vi "XY Graph Check-Uncheck Menu Items.vi"(8 "Error In":errorcluster, 10 "Menu in":refnum<k9>, 11 "XY Graph Refnum":T1) -> (0 "Error Out (dup)":errorcluster, 1 "Click Location":T2, 2 "Menu out":refnum<k9>, 3 "XY Graph Refnum dup":T1)   [LabVIEW 2021, in "XY Graph Add-Ons.lvlib"]
doc: "Check whether the Tools Panels and Grida are visible or not, and add/remove checkmarks accordingly."
uses:
  XY Graph Add-Ons.lvlib
  XY Graph Refnum.ctl
  XY Graph Click Location.ctl
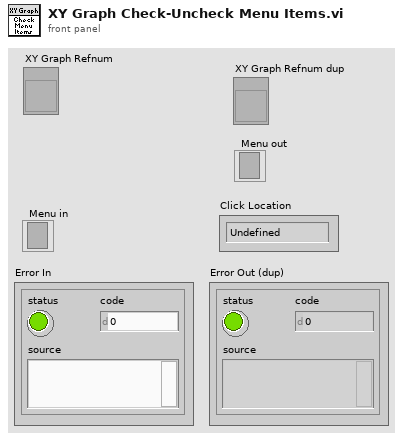
[diagram p1: front panel]
types:
  T1 = typedef "XY Graph Add-Ons.lvlib/XY Graph Refnum.ctl" = refnum<vi>
  T2 = typedef "XY Graph Add-Ons.lvlib/XY Graph Click Location.ctl" = enum16{"Undefined", "Plot Area", "Plot Legend", "Scale Legend", "Graph Palette", "Cursor Legend", "Graph Border"}
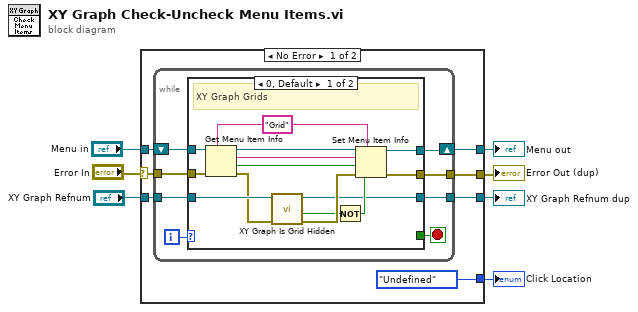
[diagram p0: block diagram]
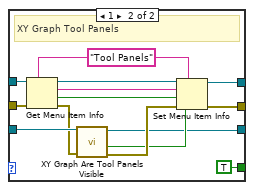
[diagram p2: hidden frame]
diagram:
  n1 = case shown="No Error" "Error In" {
    selector: "Error In" -> [w13 w53]
    tunnel: "XY Graph Refnum" -> [w12 w51]
    tunnel: "Menu in" -> [w14 w52]
    tunnel: [XY_Graph_Click_Location."Undefined" ("Click Location") _] -> w4
    tunnel: [w10 w53] -> w3
    tunnel: [w9 w52] -> w2
    tunnel: [w8 w51] -> w1
    frame No Error {
      n2 = while {
        tunnel: w12 -> [w22]
        tunnel: w13 -> [w19]
        shift-right: [w18] -> w9
        shift-left: w14 -> [w21]
        tunnel: [w16] -> w10
        tunnel: [w15] -> w8
        i -> [w20]
        stop <- w17 stop-if-true
        n3 = case shown="0, Default" w20 {
          tunnel: w22 -> [w36 w43]
          tunnel: w21 -> [w35 w50]
          tunnel: w19 -> [w33 w49]
          tunnel: [w25 w44] -> w18
          tunnel: [_ TRUE] -> w17
          tunnel: [w24 w38] -> w16
          tunnel: [w23 w37] -> w15
          frame 0, Default {
            w26 = "Grid" ("item tag")
            # "XY Graph Grids"
            n4 = Get Menu Item Info(7:w26, 8:w33, 11:w35) -> (0:w34:errorcluster, 1:w28:bool, 2:w27:string, 3:w32:refnum<k9>)  [unwired: 3 out]
            n5 = call "XY Graph Is Grid Hidden.vi"("Error In"=w34, "XY Graph Ref"=w36) -> ("Error Out (dup)"=w31:errorcluster, "Hidden Grid(s)"=w30:bool, "XY Graph Ref out"=w23:T1)  [unwired: 7 in]
            n6 = Not(x=w30) -> (.not. x?=w29:bool)
            n7 = Set Menu Item Info(6:w29, 7:w26, 8:w31, 9:w28, 10:w27, 11:w32) -> (0:w24:errorcluster, 3:w25:refnum<k9>)  [unwired: 1 in]
          }
          frame 1 {
            w45 = "Tool Panels" ("item tag")
            # "XY Graph Tool Panels"
            n8 = Get Menu Item Info(7:w45, 8:w49, 11:w50) -> (0:w42:errorcluster, 1:w47:bool, 2:w46:string, 3:w48:refnum<k9>)  [unwired: 3 out]
            n9 = call "XY Graph Are Tool Panels Visible.vi"("Error In"=w42, "XY Graph Ref"=w43) -> ("Error Out"=w41:errorcluster, "Any Panel Visible?"=w40:bool, "XY Graph Ref dup"=w37:T1)  [unwired: 6 in, 1 out]
            n10 = Set Menu Item Info(6:w40, 7:w45, 8:w41, 9:w47, 10:w46, 11:w48) -> (0:w38:errorcluster, 3:w44:refnum<k9>)  [unwired: 1 in]
          }
        }
      }
    }
    frame Error {
    }
  }
  "Error Out (dup)" <- w3
  "Click Location" <- w4
  "Menu out" <- w2
  "XY Graph Refnum dup" <- w1
